vi "tag bus to input parameters.vi"(10 "Processing Inputs":T1 {"Range"."output low" format="%.2f"; "Range"."output high" format="%.2f"}, 11 "parameter allocation":T2) -> (3 "inputs":T3)   [LabVIEW 2014, in "Tagbus PID Module runtime.lvclass"]
uses:
  Tagbus PID Module runtime.lvclass
  <vilib>/NI/Tag Bus/table/data table.ctl
  processing inputs.ctl
  <vilib>/NI/Tag Bus/table/data polymorphs/read one/read Double.vi
  <vilib>/NI/Tag Bus/table/data table.lvlib
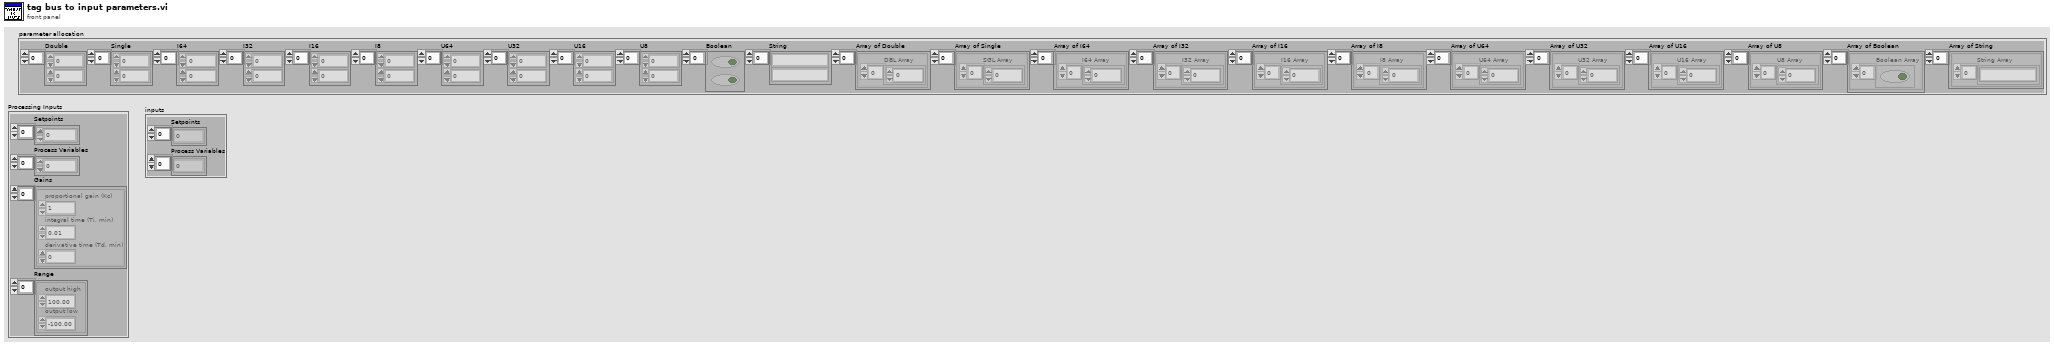
[diagram p1: front panel]
types:
  T1 = typedef "Tagbus PID Module runtime.lvclass/processing inputs.ctl" = cluster{"Setpoints":i32[], "Process Variables":i32[], "Gains":cluster{"proportional gain (Kc)":dbl, "integral time (Ti, min)":dbl, "derivative time (Td, min)":dbl}[], "Range":cluster{"output high":dbl, "output low":dbl}[]}
  T2 = typedef "tag bus.lvlib/data table.lvlib/data table.ctl" = cluster{"Double":dbl[], "Single":sgl[], "I64":i64[], "I32":i32[], "I16":i16[], "I8":i8[], "U64":u64[], "U32":u32[], "U16":u16[], "U8":u8[], "Boolean":bool[], "String":string[], "Array of Double":cluster{"DBL Array":dbl[]}[], "Array of Single":cluster{"SGL Array":sgl[]}[], "Array of I64":cluster{"I64 Array":i64[]}[], "Array of I32":cluster{"I32 Array":i32[]}[], "Array of I16":cluster{"I16 Array":i16[]}[], "Array of I8":cluster{"I8 Array":i8[]}[], "Array of U64":cluster{"U64 Array":u64[]}[], "Array of U32":cluster{"U32 Array":u32[]}[], "Array of U16":cluster{"U16 Array":u16[]}[], "Array of U8":cluster{"U8 Array":u8[]}[], "Array of Boolean":cluster{"Boolean Array":bool[]}[], "Array of String":cluster{"String Array":string[]}[]}
  T3 = cluster{"Setpoints":dbl[], "Process Variables":dbl[]}
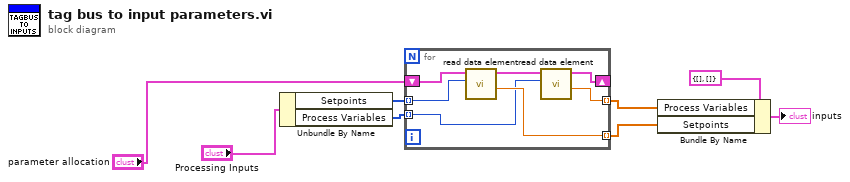
[diagram p0: block diagram]
diagram:
  n1 = Unbundle By Name("Processing Inputs") -> ("Setpoints"=w2:i32[], "Process Variables"=w4:i32[])
  n2 = for {
    tunnel: w2 -> [w15] mode=indexing
    tunnel: [w13] -> w7 mode=indexing
    shift-right: [w10] -> _
    shift-left: "parameter allocation" -> [w14]
    tunnel: w4 -> [w12] mode=indexing
    tunnel: [w9] -> w6 mode=indexing
    n3 = call-poly <vilib>:"read data element.vi"("index"=w15, "data table in"=w14) -> ("value"=w13:dbl, "data table out"=w11:T2)  [unwired: 8 in]
    n4 = call-poly <vilib>:"read data element.vi"("index"=w12, "data table in"=w11) -> ("value"=w9:dbl, "data table out"=w10:T2)  [unwired: 8 in]
  }
  n5 = Bundle By Name(cluster=T3 {"Setpoints"=[], "Process Variables"=[]} ("input cluster"), "Process Variables"=w6, "Setpoints"=w7) -> (→"inputs":T3)
